vi "Tusk.MessageAllSenderCore.vi"(5 "Priority?":bool, 8 "error in (no error)":errorcluster, 10 "Message":refnum<class "Message.lvclass">, 11 "Tusk in":refnum<class "Tusk.lvclass">) -> (0 "error out":errorcluster, 3 "Tusk out":refnum<class "Tusk.lvclass">)   [LabVIEW 2018, in "Application.lvlib" / "Tusk.lvclass"]
uses:
  Tusk.lvclass
  Message Class/Message.lvclass
  Tusk.lvclass/Tusk.ctl
  Dictionary Class/Dictionary.lvclass/Dictionary.ctl
  1679c56e-e765-44f0-aff8-f47c4dbf3d60.vi
  Dictionary Class/VIs/Get Data DVR.vi
  Exceptions Class/VIs/Invalid Type.vi
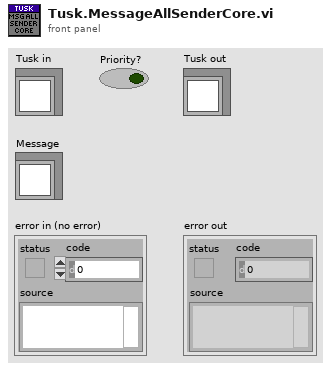
[diagram p1: front panel]
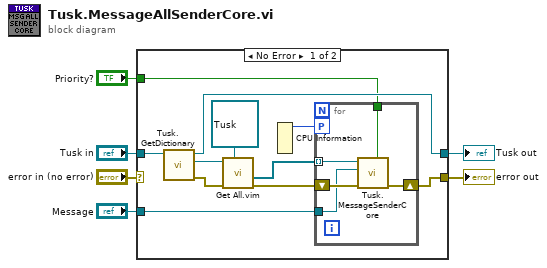
[diagram p0: block diagram]
diagram:
  n1 = case shown="No Error" "error in (no error)" {
    selector: "error in (no error)" -> [_ w24]
    tunnel: [w7 w24] -> w5
    tunnel: [w17 w23] -> w3
    tunnel: "Tusk in" -> [w16 w23]
    tunnel: "Priority?" -> [w11 _]
    tunnel: "Message" -> [w10 _]
    frame No Error {
      n2 = call "Tusk.GetDictionary.vi"("Tusk in"=w16) -> ("error out"=w13:errorcluster, "Dictionary"=w15:refnum<class "Dictionary.lvclass">, "Tusk out"=w17:refnum<class "Tusk.lvclass">)  [unwired: 8 in]
      n3 = call "Get All.vim"("Base Type"=refnum<class "Tusk.lvclass"> refnum ("Tusk out"), "error in (no error)"=w13, "Dictionary in"=w15) -> ("error out"=w8:errorcluster, "Values"=w12:refnum<class "Tusk.lvclass">[])  [unwired: 5 in, 2 out]
      n4 = CPU Information() -> (4:w9:i32)  [unwired: 3 out]
      n5 = for {
        tunnel: w12 -> [w22] mode=indexing
        tunnel: w11 -> [w21]
        tunnel: w10 -> [w19]
        workers-P: w9 -> [_]
        shift-right: [w18] -> w7
        shift-left: w8 -> [w20]
        n6 = call "Tusk.MessageSenderCore.vi"("Priority?"=w21, "error in (no error)"=w20, "Message"=w19, "Tusk in"=w22) -> ("error out"=w18:errorcluster)  [unwired: 5 in, 2 out]
      }
    }
    frame Error {
    }
  }
  "error out" <- w5
  "Tusk out" <- w3
